vi "init.vi"(8 "error in":errorcluster, 10 "TBM module configuration in":refnum<class "TBM module configuration.lvclass">, 11 "tag select module runtime in":refnum<class "tag select module runtime.lvclass">) -> (0 "error out":errorcluster, 1 "data allocations":T1, 2 "execution settings":T4, 3 "tag select module runtime out":refnum<class "tag select module runtime.lvclass">)   [LabVIEW 2013, in "tag select module runtime.lvclass"]
doc: "Provides an interface for initializing a module at runtime. While this interface performs no operations, a child should provide an override which may open any necessary references or sessions, allocate necessary memory, and perform any final configuration validataion before providing the full configuration <b>execution data</b> to the calling process."
uses:
  tag select module runtime.lvclass
  <vilib>/NI/Tag Bus Module Framework/channel/TBM channel.lvclass
  <vilib>/NI/Tag Bus Module Framework/runtime/TBM module execution interface.lvclass
  configuration/tag select module configuration.lvclass
  <vilib>/NI/Tag Bus Module Framework/module configuration/TBM module configuration.lvclass
  <vilib>/NI/Tag Bus Module Framework/runtime/execution settings.ctl
  <vilib>/NI/Tag Bus Module Framework/channel/data tables.ctl
  <vilib>/NI/Tag Bus/dictionary/data dictionary.lvclass
  <vilib>/NI/Tag Bus/dictionary table pair.ctl
  <vilib>/NI/Tag Bus/tag bus.lvlib
  <vilib>/NI/Tag Bus/table/data table.ctl
  <vilib>/NI/Tag Bus/table/data table.lvlib
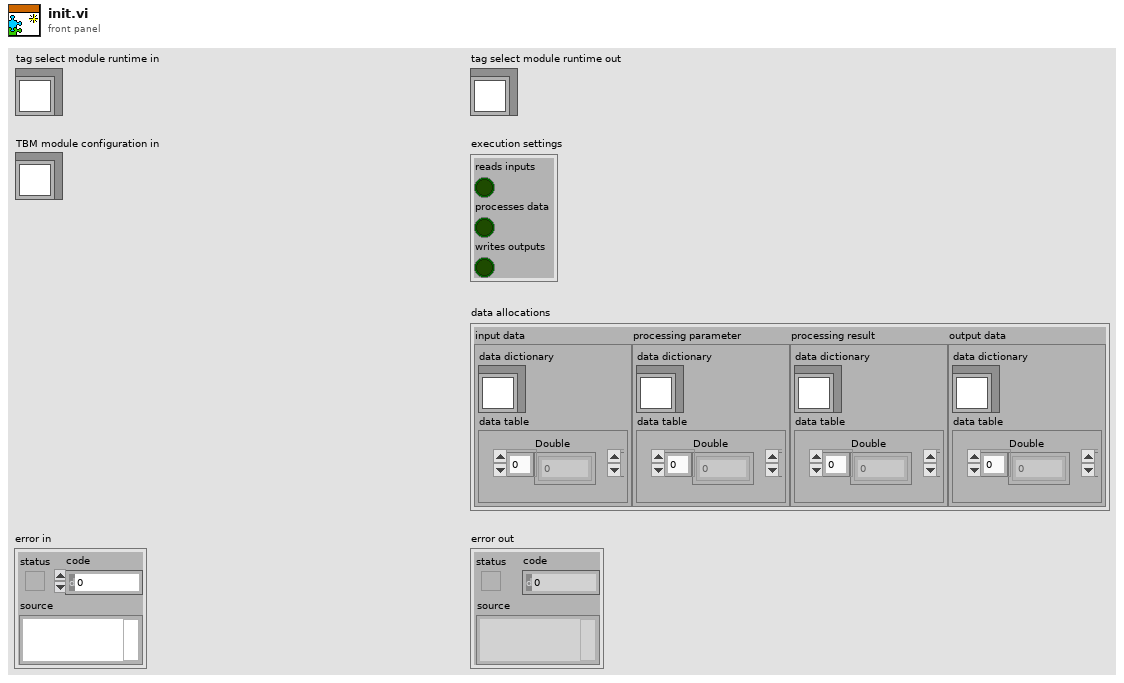
[diagram p1: front panel]
types:
  T1 = typedef "TBM channel.lvclass/data tables.ctl" = cluster{"input data":T2, "processing parameter":T2, "processing result":T2, "output data":T2}
  T2 = typedef "tag bus.lvlib/dictionary table pair.ctl" = cluster{"data dictionary":refnum<class "data dictionary.lvclass">, "data table":T3}
  T3 = typedef "tag bus.lvlib/data table.lvlib/data table.ctl" = cluster{"Double":dbl[], "Single":sgl[], "I64":i64[], "I32":i32[], "I16":i16[], "I8":i8[], "U64":u64[], "U32":u32[], "U16":u16[], "U8":u8[], "Boolean":bool[], "String":string[], "Array of Double":cluster{"DBL Array":dbl[]}[], "Array of Single":cluster{"SGL Array":sgl[]}[], "Array of I64":cluster{"I64 Array":i64[]}[], "Array of I32":cluster{"I32 Array":i32[]}[], "Array of I16":cluster{"I16 Array":i16[]}[], "Array of I8":cluster{"I8 Array":i8[]}[], "Array of U64":cluster{"U64 Array":u64[]}[], "Array of U32":cluster{"U32 Array":u32[]}[], "Array of U16":cluster{"U16 Array":u16[]}[], "Array of U8":cluster{"U8 Array":u8[]}[], "Array of Boolean":cluster{"Boolean Array":bool[]}[], "Array of String":cluster{"String Array":string[]}[]}
  T4 = typedef "TBM module execution interface.lvclass/execution settings.ctl" = cluster{"reads inputs":bool, "processes data":bool, "writes outputs":bool}
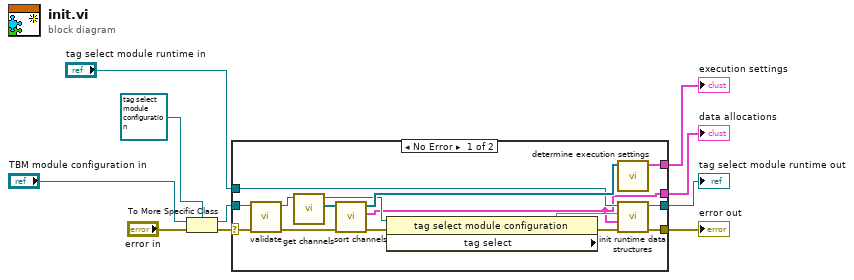
[diagram p0: block diagram]
diagram:
  n1 = To More Specific Class(target class=refnum<class "tag select module configuration.lvclass"> refnum ("Synchronous module configuration"), reference="TBM module configuration in", error in="error in") -> (specific class reference=w9:refnum<class "tag select module configuration.lvclass">, error out=w10:errorcluster)
  n2 = case shown="No Error" w10 {
    selector: w10 -> [w21 w26]
    tunnel: w9 -> [w20 _]
    tunnel: "tag select module runtime in" -> [w14 w27]
    tunnel: [w13 w27] -> w4
    tunnel: [w16 w26] -> w3
    tunnel: [w11 _] -> w1
    tunnel: [w24 _] -> w2
    frame No Error {
      n3 = call-dynamic "validate.vi"("error in"=w21, "tag select module configuration in"=w20) -> ("error out"=w22:errorcluster, "tag select module configuration out"=w19:refnum<class "tag select module configuration.lvclass">)  [unwired: 8 in]
      n4 = call-dynamic "get channels.vi"("tag select module configuration in"=w19) -> ("channels"=w18:refnum<class "TBM channel.lvclass">[], "tag select module configuration out"=w17:refnum<class "tag select module configuration.lvclass">)  [unwired: 9 in]
      n5 = call <vilib>:"sort channels.vi"("error in"=w22, "channels in"=w18) -> ("error out"=w25:errorcluster, "data allocations"=w11:T1, "channels out"=w23:refnum<class "TBM channel.lvclass">[])  [unwired: 7 in]
      n6 = property class="tag select module configuration"(reference=w17, error in=w25) -> (error out=w15:errorcluster, "tag select"=w12)  [unwired: 1 out]
      n7 = call <vilib>:"determine execution settings.vi"("channels"=w23) -> ("execution settings"=w24:T4)  [unwired: 10 in]
      n8 = call "init runtime data structures.vi"("error in"=w15, "data allocations"=w11, "tag select"=w12, "tag select module runtime in"=w14) -> ("error out"=w16:errorcluster, "tag select module runtime out"=w13:refnum<class "tag select module runtime.lvclass">)  [unwired: 6 in]
    }
    frame Error {
    }
  }
  "error out" <- w3
  "tag select module runtime out" <- w4
  "execution settings" <- w2
  "data allocations" <- w1
